vi "Update Position.vi"(0 "Last Position X":dbl, 1 "Initial Yaw":dbl=90.0, 5 "Last Postion Y":dbl, 7 "Last Postion Z":dbl, 9 "Last Left Dist":dbl, 11 "Last Right Dist":dbl) -> (4 "New X":dbl, 6 "New Y":dbl, 8 "New Z":dbl, 10 "Left Dist Travelled Out (cm)":dbl, 15 "Right Dist Travelled Out (cm)":dbl)   [LabVIEW 2009]
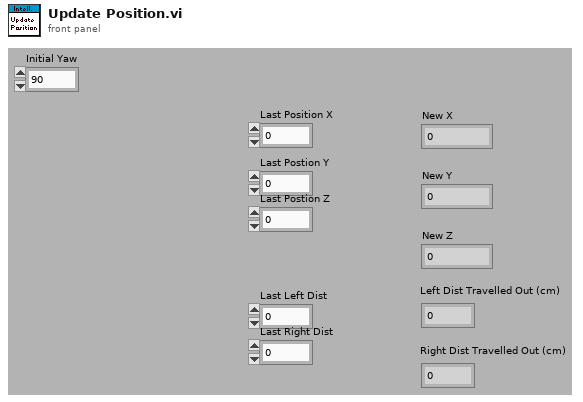
[diagram p1: front panel]
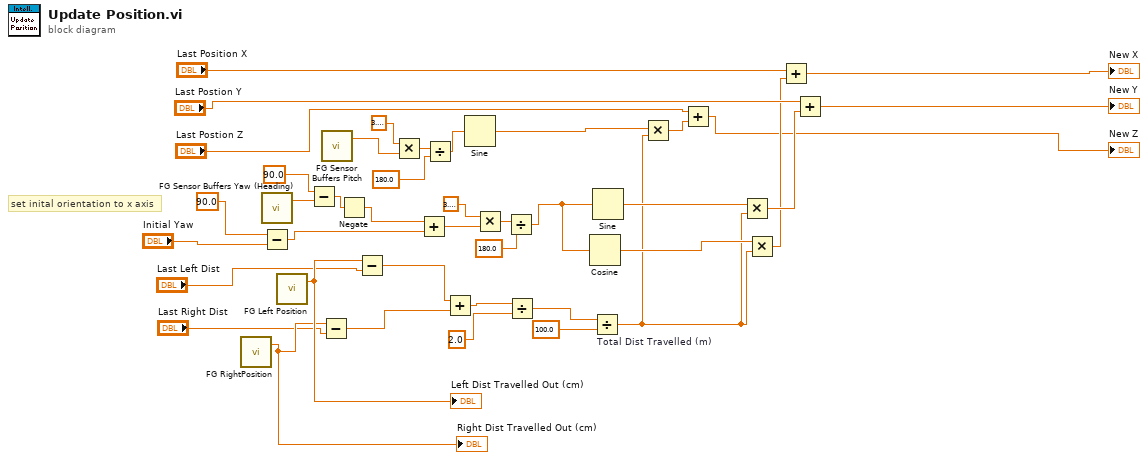
[diagram p0: block diagram]
diagram:
  # "set inital orientation to x axis"
  n1 = call "FG RightPosition.vi"() -> ("Right Dist Travelled Out (cm)"=w13:dbl)  [unwired: 3 in]
  "Right Dist Travelled Out (cm)" <- w13
  n2 = call "FG Sensor Buffers Yaw (Heading).vi"() -> ("Yaw Buffer Out"=w3:dbl)  [unwired: 3 in]
  n3 = Subtract(x=90.0 ("y"), y="Initial Yaw") -> (x-y=w5:dbl)
  n4 = call "FG Left Position.vi"() -> ("Left Dist Travelled Out (cm)"=w15:dbl)  [unwired: 3 in]
  "Left Dist Travelled Out (cm)" <- w15
  n5 = Subtract(x=90.0 ("y"), y=w3) -> (x-y=w2:dbl)
  n6 = Subtract(x=w13, y="Last Right Dist") -> (x-y=w17:dbl)
  n7 = call "FG Sensor Buffers Pitch.vi"() -> ("Pitch Buffer out"=w28:dbl)  [unwired: 3 in]
  n8 = Negate(x=w2) -> (-x=w1:dbl)
  n9 = Subtract(x=w15, y="Last Left Dist") -> (x-y=w18:dbl)
  n10 = Multiply(x=3.141592653589793, y=w28) -> (x*y=w25:dbl)
  n11 = Add(x=w1, y=w5) -> (x+y=w20:dbl)
  n12 = Divide(x=w25, y=180.0) -> (x/y=w26:dbl)
  n13 = Add(x=w18, y=w17) -> (x+y=w35:dbl)
  n14 = Sine(x=w26) -> (sin(x)=w11:dbl)
  n15 = Multiply(x=3.141592653589793, y=w20) -> (x*y=w22:dbl)
  n16 = Divide(x=w22, y=180.0) -> (x/y=w19:dbl)
  n17 = Divide(x=w35, y=2.0) -> (x/y=w33:dbl)
  n18 = Cosine(x=w19) -> (cos(x)=w31:dbl)
  n19 = Divide "Total Dist Travelled (m)"(x=w33, y=100.0) -> (x/y=w16:dbl)
  n20 = Sine(x=w19) -> (sin(x)=w32:dbl)
  n21 = Multiply(x=w11, y=w16) -> (x*y=w9:dbl)
  n22 = Add(x="Last Postion Z", y=w9) -> (x+y=→"New Z":dbl)
  n23 = Multiply(x=w32, y=w16) -> (x*y=w30:dbl)
  n24 = Multiply(x=w31, y=w16) -> (x*y=w29:dbl)
  n25 = Add(x="Last Position X", y=w29) -> (x+y=→"New X":dbl)
  n26 = Add(x="Last Postion Y", y=w30) -> (x+y=→"New Y":dbl)
